vi "Configure Measurement Input Connector.vi"(8 "error in (no error)":errorcluster, 9 "Input Connector (\"\")":string, 10 "Instance (1)":i32=1, 11 "VISA resource name":refnum<visa-resource-name>) -> (0 "error out":errorcluster, 3 "VISA resource name out":refnum<visa-resource-name>)   [LabVIEW 2020, in "Rohde&Schwarz CMXP GPRF.lvlib"]
doc: "Selects the input connector for the measured signal.\n\nAttribute:\nRSCMXPGPRF_ATTR_MEASUREMENT_INPUT_CONNECTOR\n\nRemote-control command:\nROUTe:GPRF:MEAS<i>:SPATh"
uses:
  <instrlib>/Rohde&Schwarz CMXP GPRF/Rohde&Schwarz CMXP GPRF.lvlib
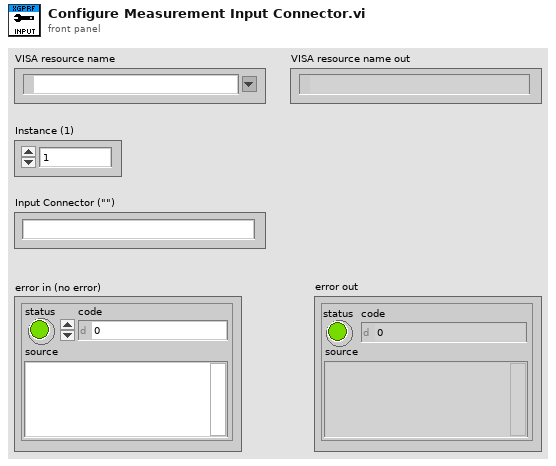
[diagram p1: front panel]
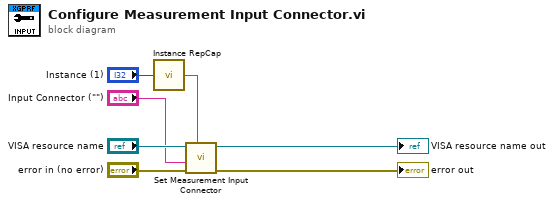
[diagram p0: block diagram]
diagram:
  n1 = call <instrlib>:"Instance RepCap.vi"("Instance in"="Instance (1)") -> ("Instance out"=w2:string)
  n2 = call "Set Measurement Input Connector"("Repeated Capabilities"=w2, "error in (no error)"="error in (no error)", "Measurement Input Connector ()"="Input Connector (\"\")", "instrument handle"="VISA resource name") -> ("error out"=→"error out":errorcluster, "instrument handle out"=→"VISA resource name out":refnum<visa-resource-name>)  [unwired: 6 in]
